vi "MICS Dongle Interface.vi"() -> ()   [LabVIEW 2010]
uses:
  <vilib>/Instr/_visa.llb/VISA Configure Serial Port (Instr).vi
panel:
  out "Reply Hex Data":string
  in  "Write Data":T1 {"Pack Data" format="%02x"}
  out "Output Numeric":u8[](array[numeric]) format="%02x"
  in  "stop":bool
  in  "R/W Delay":u32=200
  in  "VISA resource name":refnum<visa-resource-name>
  in  "OK Button":bool
  out "Reply Text":string
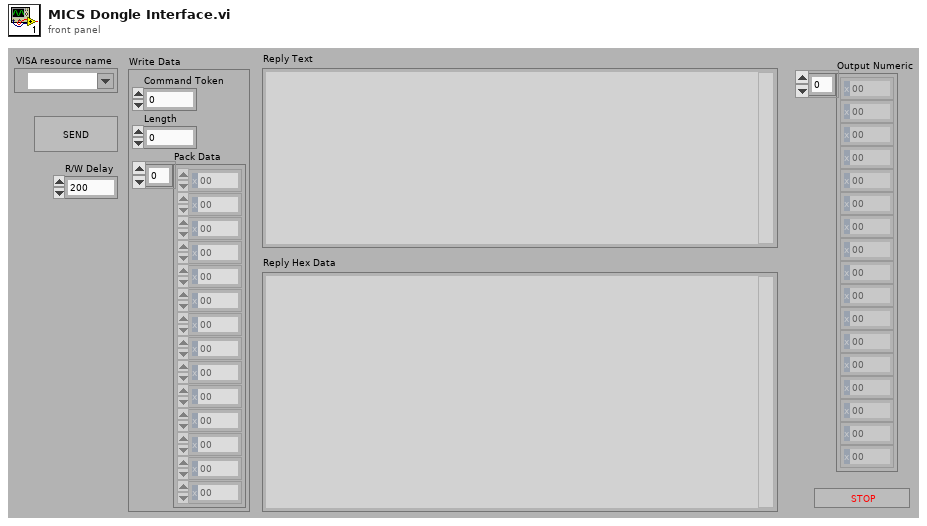
[diagram p1: front panel]
types:
  T1 = cluster{"Command Token":u8, "Length":u16, "Pack Data":u8[]}
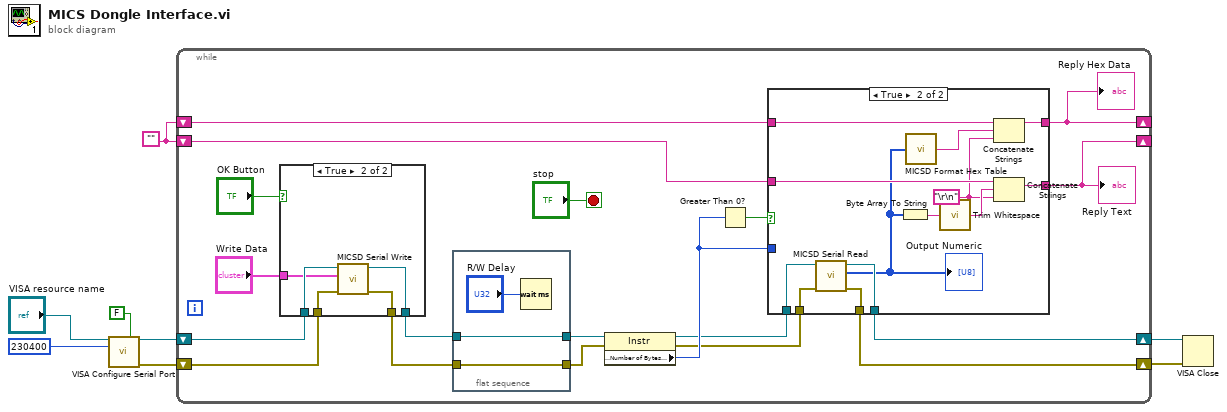
[diagram p0: block diagram]
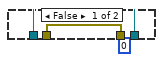
[diagram p3: hidden frame]
diagram:
  w2 = ""
  n1 = call-poly "VISA Configure Serial Port"("VISA resource name"="VISA resource name", "Enable Termination\nChar (T)"=FALSE ("Enable Termination\nChar (T)"), "baud rate (9600)"=u32 230400) -> ("VISA resource name out"=w7:refnum<visa-resource-name>, "error out"=w6:errorcluster)  [unwired: 11 in]
  n2 = while {
    shift-right: [w12] -> w5
    shift-left: w7 -> [w26]
    shift-right: [w13] -> w4
    shift-left: w6 -> [w25]
    shift-right: [w15] -> _
    shift-left: w2 -> [w16]
    shift-right: [w9] -> _
    shift-left: w2 -> [w10]
    stop <- "stop" stop-if-true
    n3 = case shown="True" "OK Button" {
      tunnel: w26 -> [w49 w53]
      tunnel: w25 -> [w48 w54]
      tunnel: [w48 w52] -> w24
      tunnel: [w49 w51] -> w23
      tunnel: "Write Data" -> [_ w50]
      frame False {
        (unwired) u32 0 ("return count")
      }
      frame True {
        n4 = call "MICSD Serial Write.vi"("error in (no error)"=w54, "Write Data"=w50, "VISA Resource Name"=w53) -> ("error out"=w52:errorcluster, "DUP Visa Resource Name"=w51:refnum<visa-resource-name>)  [unwired: 7 in]
      }
    }
    n5 = flat-sequence {
      tunnel: w24 -> [w45]
      tunnel: w23 -> [w46]
      tunnel: [w46] -> w22
      tunnel: [w45] -> w21
      frame #0 {
        n6 = Wait (ms)(milliseconds to wait="R/W Delay") -> ()  [unwired: 1 out]
      }
    }
    n7 = property class="Instr"(reference=w22, error in=w21) -> (reference out=w18:refnum<visa-resource-name>, error out=w17:errorcluster, "Serial Settings:Number of Bytes at Serial Port"=w19:u32)
    n8 = Greater Than 0?(x=w19) -> (x > 0?=w20:bool)
    n9 = case shown="True" w20 {
      tunnel: w16 -> [w31 w44]
      tunnel: w19 -> [_ _]
      tunnel: w17 -> [w30 w42]
      tunnel: w18 -> [w29 w41]
      tunnel: [w31 w43] -> w15
      tunnel: [w30 w40] -> w13
      tunnel: [w29 w39] -> w12
      tunnel: w10 -> [w28 w35]
      tunnel: [w28 w34] -> w9
      frame False {
      }
      frame True {
        w32 = "\r\n"
        n10 = call "MICSD Serial Read.vi"("error in (no error)"=w42, "VISA Resource Name"=w41) -> ("error out"=w40:errorcluster, "Read Data"=w37:u8[], "DUP Visa Resource Name"=w39:refnum<visa-resource-name>)  [unwired: 7 in]
        "Output Numeric" <- w37
        n11 = Byte Array To String(unsigned byte array=w37) -> (string=w38:string)
        n12 = call "MICSD Format Hex Table.vi"("Read Data"=w37) -> ("String"=w36:string)  [unwired: 4 in]
        n13 = call <vilib>:"Trim Whitespace.vi"("string"=w38) -> ("trimmed string"=w33:string)  [unwired: 1 in]
        n14 = Concatenate Strings(w35, w36, w32) -> (w34:string)
        n15 = Concatenate Strings(w44, w33, w32) -> (w43:string)
      }
    }
    "Reply Text" <- w15
    "Reply Hex Data" <- w9
  }
  n16 = VISA Close(VISA resource name=w5, error in (no error)=w4) -> ()  [unwired: 1 out]
